vi "Setup For Triggered Images v4.2Test.vi"(4 "error in":errorcluster caption="error in (no error)", 5 "Timeout (ms)":u32=1000, 6 "Gain":dbl, 7 "Shutter speed":dbl, 8 "Camera Name":T3) -> (0 "Error out":errorcluster caption="error in (no error)", 1 "Session Out":T3)   [LabVIEW 2013]
doc: "The Grab and Attributes Setup VI acquires images continuously and displays the images in an image control using high-level acquisition VIs. The VI also modifes the camera attributes while acquiring images. A grab is appropriate for high-speed applications in which you need to process only one image at a time."
uses:
  <vilib>/userdefined/High Color/IMAQdx.ctl
  <vilib>/vision/driver/IMAQdx.llb/IMAQdx Attribute Type.ctl
  <vilib>/vision/driver/IMAQdx.llb/IMAQdx Attribute Visibility.ctl
  <vilib>/vision/driver/IMAQdx.llb/IMAQdx Acquisition Mode.ctl
  <vilib>/vision/driver/NI_Vision_Acquisition_Software.lvlib
  <resource>/objmgr/imaqdx.rc
panel:
  out "Width":u32
  out "Attribute Information Array":T2(array[cluster])
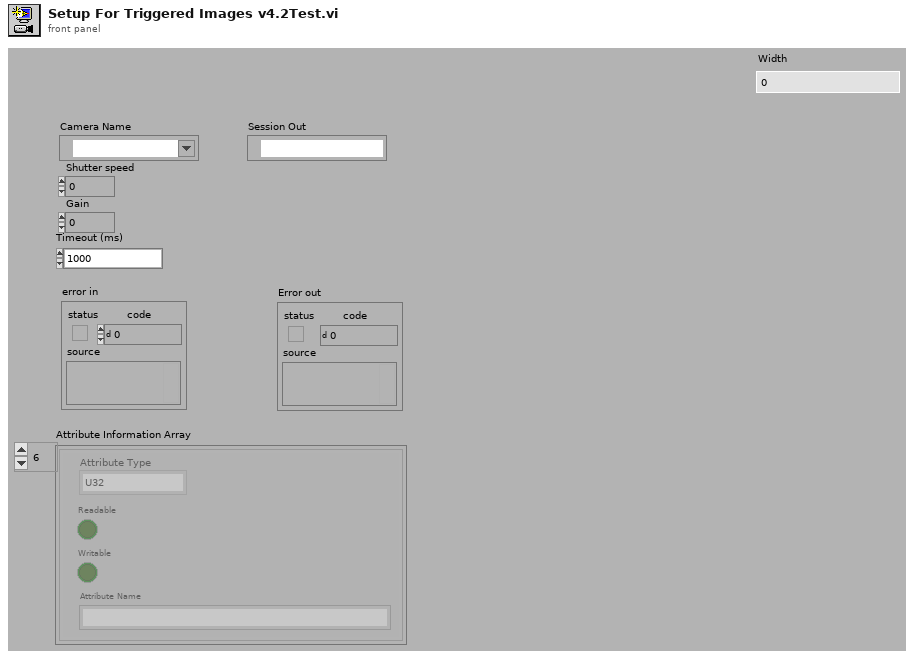
[diagram p1: front panel]
types:
  T1 = typedef "NI_Vision_Acquisition_Software.lvlib/IMAQdx Attribute Type.ctl" = enum32{"U32", "I64", "DBL", "String", "Enum", "Bool", "Command"}
  T2 = cluster{"Attribute Type":T1, "Readable":bool, "Writable":bool, "Attribute Name":string}[]
  T3 = typedef "IMAQdx.ctl" = refnum<k21>
  T4 = typedef "NI_Vision_Acquisition_Software.lvlib/IMAQdx Attribute Visibility.ctl" = enum32{"Simple", "Intermediate", "Advanced"}
  T5 = typedef "NI_Vision_Acquisition_Software.lvlib/IMAQdx Acquisition Mode.ctl" = enum32{"One Shot", "Continuous"}
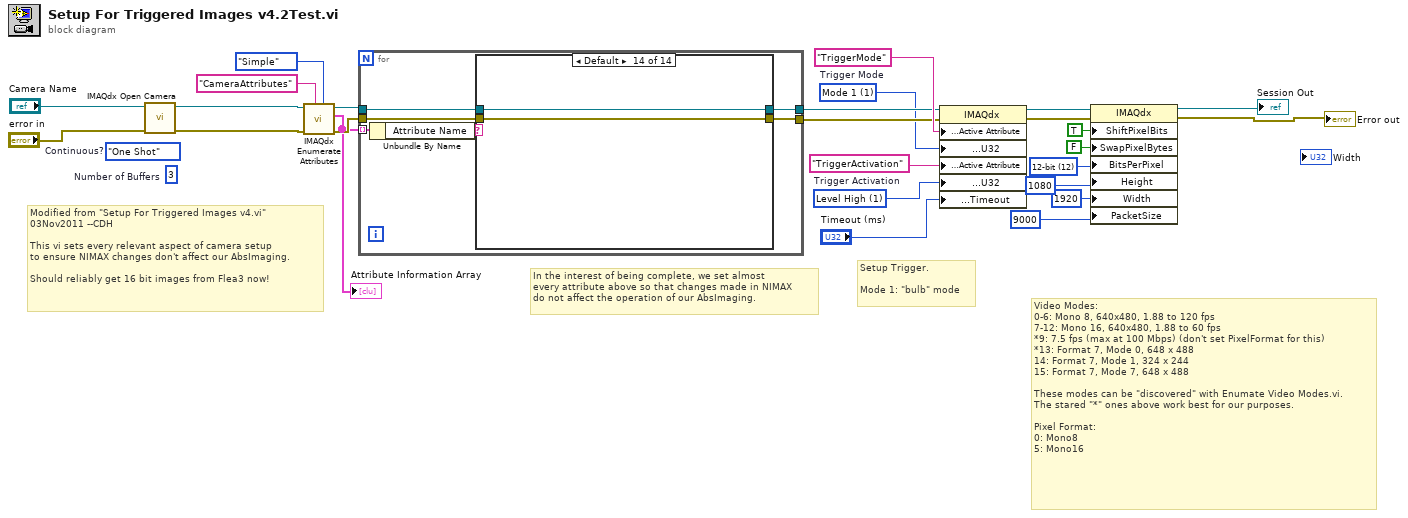
[diagram p0: block diagram]
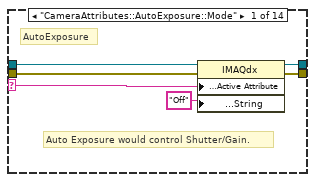
[diagram p2: hidden frame]
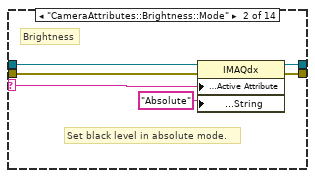
[diagram p3: hidden frame]
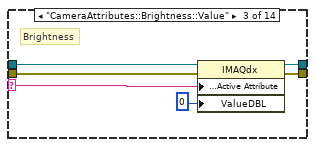
[diagram p4: hidden frame]
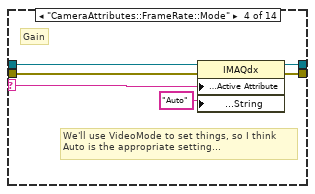
[diagram p5: hidden frame]
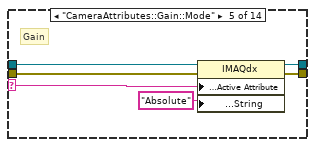
[diagram p6: hidden frame]
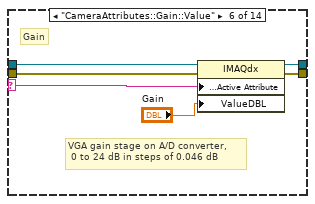
[diagram p7: hidden frame]
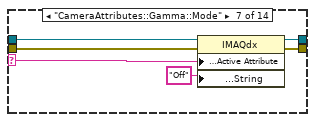
[diagram p8: hidden frame]
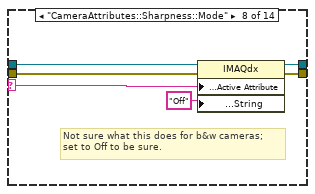
[diagram p9: hidden frame]
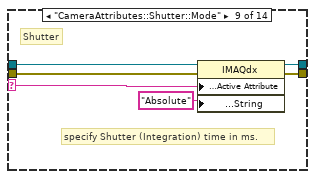
[diagram p10: hidden frame]
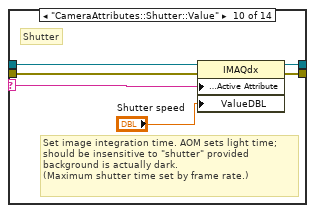
[diagram p11: hidden frame]
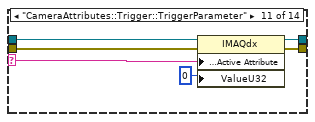
[diagram p12: hidden frame]
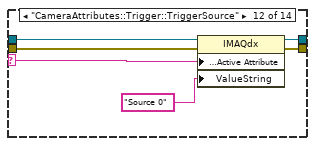
[diagram p13: hidden frame]
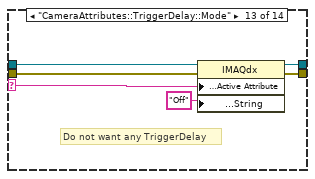
[diagram p14: hidden frame]
diagram:
  w4 = u32 12 items=["Use Hardware Value"=0, "10-bit"=10, "12-bit"=12, "14-bit"=14, "16-bit"=16] ("BitsPerPixel")
  w17 = u32 1 items=["Mode 0"=0, "Mode 1"=1, "Mode 3"=3, "Mode 14"=14, "Mode 15"=15, "Off"=16]  # Trigger Mode
  w16 = u32 1 items=["Level Low", "Level High"]  # Trigger Activation
  (unwired) u32 3  # Number of Buffers
  (unwired) IMAQdx_Acquisition_Mode."One Shot"  # Continuous?
  # "Modified from \"Setup For Triggered Images v4.vi\"\n03Nov2011 --CDH\n\nThis vi sets every relevant aspect of camera setup\nto ensure NIMAX changes don't affect our AbsImaging.\n\nShould reliably get 16 bit images from Flea3 now!"
  # "In the interest of being complete, we set almost\nevery attribute above so that changes made in NIMAX\ndo not affect the operation of our AbsImaging."
  # "Video Modes:\n0-6: Mono 8, 640x480, 1.88 to 120 fps\n7-12: Mono 16, 640x480, 1.88 to 60 fps\n*9: 7.5 fps (max at 100 Mbps) (don't set PixelFormat for this)\n*13: Format 7, Mode 0, 648 x 488\n14: Format 7, Mode 1, 324 x 244\n15: Format 7, Mode 7, 648 x 488 \n\nThese modes can be \"discovered\" with Enumate Video Modes.vi.\nThe stared \"*\" ones above work best for our purposes.\n\nPixel Format:\n0: Mono8\n5: Mono16"
  # "Setup Trigger.\n\nMode 1: \"bulb\" mode"
  n1 = call <vilib>:"IMAQdx Open Camera.vi"("error in"="error in", "Session In"="Camera Name") -> ("error out"=w13:errorcluster, "Session Out"=w14:T3)  [unwired: 1 in, 7 out]
  n2 = call <vilib>:"IMAQdx Enumerate Attributes.vi"("Visibility"=IMAQdx_Attribute_Visibility."Simple", "Root"="CameraAttributes", "error in"=w13, "Session In"=w14) -> ("error out"=w26:errorcluster, "Attribute Information Array"=w22:T2, "Session Out"=w25:T3)  [unwired: 5 out]
  "Attribute Information Array" <- w22
  n3 = for {
    tunnel: w22 -> [w32] mode=indexing
    tunnel: w25 -> [w31]
    tunnel: w26 -> [w30]
    tunnel: [w28] -> w19
    tunnel: [w27] -> w18
    n4 = Unbundle By Name(w32) -> ("Attribute Name"=w29:string)
    n5 = case shown="Default" w29 {
      selector: w29 -> [w34 w40 w46 w52 w58 w64 w70 w76 w82 w88 w94 w100 w106 _]
      tunnel: w31 -> [w38 w44 w50 w56 w62 w68 w74 w80 w86 w92 w98 w104 w110 w112]
      tunnel: w30 -> [w37 w43 w49 w55 w61 w67 w73 w79 w85 w91 w97 w103 w109 w111]
      tunnel: [w36 w42 w48 w54 w60 w66 w72 w78 w84 w90 w96 w102 w108 w112] -> w28
      tunnel: [w35 w41 w47 w53 w59 w65 w71 w77 w83 w89 w95 w101 w107 w111] -> w27
      frame "CameraAttributes::AutoExposure::Mode" {
        # "Auto Exposure would control Shutter/Gain."
        # "AutoExposure"
        n6 = property class="IMAQdx"(reference=w38, error in=w37, "Camera Attributes:Active Attribute"=w34, "Camera Attributes:Value:String"="Off" ("ValueString")) -> (reference out=w36:T3, error out=w35:errorcluster)
      }
      frame "CameraAttributes::Brightness::Mode" {
        # "Set black level in absolute mode."
        # "Brightness"
        n7 = property class="IMAQdx"(reference=w44, error in=w43, "Camera Attributes:Active Attribute"=w40, "Camera Attributes:Value:String"="Absolute" ("ValueString")) -> (reference out=w42:T3, error out=w41:errorcluster)
      }
      frame "CameraAttributes::Brightness::Value" {
        # "Brightness"
        n8 = property class="IMAQdx"(reference=w50, error in=w49, "Camera Attributes:Active Attribute"=w46, "ValueDBL"=0) -> (reference out=w48:T3, error out=w47:errorcluster)
      }
      frame "CameraAttributes::FrameRate::Mode" {
        # "We'll use VideoMode to set things, so I think\nAuto is the appropriate setting..."
        # "Gain"
        n9 = property class="IMAQdx"(reference=w56, error in=w55, "Camera Attributes:Active Attribute"=w52, "Camera Attributes:Value:String"="Auto" ("ValueString")) -> (reference out=w54:T3, error out=w53:errorcluster)
      }
      frame "CameraAttributes::Gain::Mode" {
        # "Gain"
        n10 = property class="IMAQdx"(reference=w62, error in=w61, "Camera Attributes:Active Attribute"=w58, "Camera Attributes:Value:String"="Absolute" ("ValueString")) -> (reference out=w60:T3, error out=w59:errorcluster)
      }
      frame "CameraAttributes::Gain::Value" {
        # "VGA gain stage on A/D converter,\n 0 to 24 dB in steps of 0.046 dB"
        # "Gain"
        n11 = property class="IMAQdx"(reference=w68, error in=w67, "Camera Attributes:Active Attribute"=w64, "ValueDBL"="Gain") -> (reference out=w66:T3, error out=w65:errorcluster)
      }
      frame "CameraAttributes::Gamma::Mode" {
        n12 = property class="IMAQdx"(reference=w74, error in=w73, "Camera Attributes:Active Attribute"=w70, "Camera Attributes:Value:String"="Off" ("ValueString")) -> (reference out=w72:T3, error out=w71:errorcluster)
      }
      frame "CameraAttributes::Sharpness::Mode" {
        # "Not sure what this does for b&w cameras;\nset to Off to be sure."
        n13 = property class="IMAQdx"(reference=w80, error in=w79, "Camera Attributes:Active Attribute"=w76, "Camera Attributes:Value:String"="Off" ("ValueString")) -> (reference out=w78:T3, error out=w77:errorcluster)
      }
      frame "CameraAttributes::Shutter::Mode" {
        # "specify Shutter (Integration) time in ms."
        # "Shutter"
        n14 = property class="IMAQdx"(reference=w86, error in=w85, "Camera Attributes:Active Attribute"=w82, "Camera Attributes:Value:String"="Absolute" ("ValueString")) -> (reference out=w84:T3, error out=w83:errorcluster)
      }
      frame "CameraAttributes::Shutter::Value" {
        # "Set image integration time. AOM sets light time;\nshould be insensitive to \"shutter\" provided \nbackground is actually dark.\n(Maximum shutter time set by frame rate.)"
        # "Shutter"
        n15 = property class="IMAQdx"(reference=w92, error in=w91, "Camera Attributes:Active Attribute"=w88, "ValueDBL"="Shutter speed") -> (reference out=w90:T3, error out=w89:errorcluster)
      }
      frame "CameraAttributes::Trigger::TriggerParameter" {
        n16 = property class="IMAQdx"(reference=w98, error in=w97, "Camera Attributes:Active Attribute"=w94, "ValueU32"=u32 0) -> (reference out=w96:T3, error out=w95:errorcluster)
      }
      frame "CameraAttributes::Trigger::TriggerSource" {
        n17 = property class="IMAQdx"(reference=w104, error in=w103, "Camera Attributes:Active Attribute"=w100, "ValueString"="Source 0") -> (reference out=w102:T3, error out=w101:errorcluster)
      }
      frame "CameraAttributes::TriggerDelay::Mode" {
        # "Do not want any TriggerDelay"
        n18 = property class="IMAQdx"(reference=w110, error in=w109, "Camera Attributes:Active Attribute"=w106, "Camera Attributes:Value:String"="Off" ("ValueString")) -> (reference out=w108:T3, error out=w107:errorcluster)
      }
      frame Default {
      }
    }
  }
  n19 = property class="IMAQdx"(reference=w19, error in=w18, "Camera Attributes:Active Attribute"="TriggerMode" ("ActiveAttribute"), "Camera Attributes:Value:U32"=w17, "Camera Attributes:Active Attribute"="TriggerActivation" ("ActiveAttribute"), "Camera Attributes:Value:U32"=w16, "Acquisition Attributes:Timeout"="Timeout (ms)") -> (reference out=w10:T3, error out=w9:errorcluster)
  n20 = property class="IMAQdx"(reference=w10, error in=w9, "ShiftPixelBits"=TRUE, "SwapPixelBytes"=FALSE, "BitsPerPixel"=w4, "Height"=u32 1080, "Width"=u32 1920, "PacketSize"=u32 9000) -> (reference out=→"Session Out":T3, error out=→"Error out":errorcluster)
